vi "Shape Filter.vi"(11 "Image In":T1) -> (2 "Line Cam Obstacles":cluster{dbl[], dbl[], i32}, 3 "Image (out)":T1)   [LabVIEW 2011]
uses:
  <vilib>/vision/Pattern Matching.llb/IMAQ Curve Parameters.ctl
  <vilib>/vision/Analysis.llb/IMAQ ExtractCurvesCurve.ctl
  <vilib>/vision/Image Controls.llb/IMAQ Image.ctl
  <vilib>/vision/NI_Vision_Development_Module.lvlib
panel:
  out "Intensity Graph":dbl[][](graph)
  out "Curves":T2[](array[typedef]) {"Points"."Y" format="%.2f"; "Points"."X" format="%.2f"}
  out "Image out":T1(plugin-control)
  in  "Curve Parameters":T3={"Extraction Mode"=0, "Edge Threshold"=75, "Edge Filter Size"=1, "Min Length"=25, "Row Search Step Size"=15, "Col Search Step Size"=15, "Max Endpoint Gap"=10, "Closed"=FALSE, "Subpixel"=FALSE} {"Extraction Mode" items=["Normal", "Uniform Regions"]; "Edge Filter Size" items=["Fine", "Normal", "Contour Tracing"]; "Max Endpoint Gap" min=0; "Col Search Step Size" min=1 max=255 step=1; "Row Search Step Size" min=1 max=255 step=1; "Min Length" min=0; "Edge Threshold" min=1 max=350 step=1}
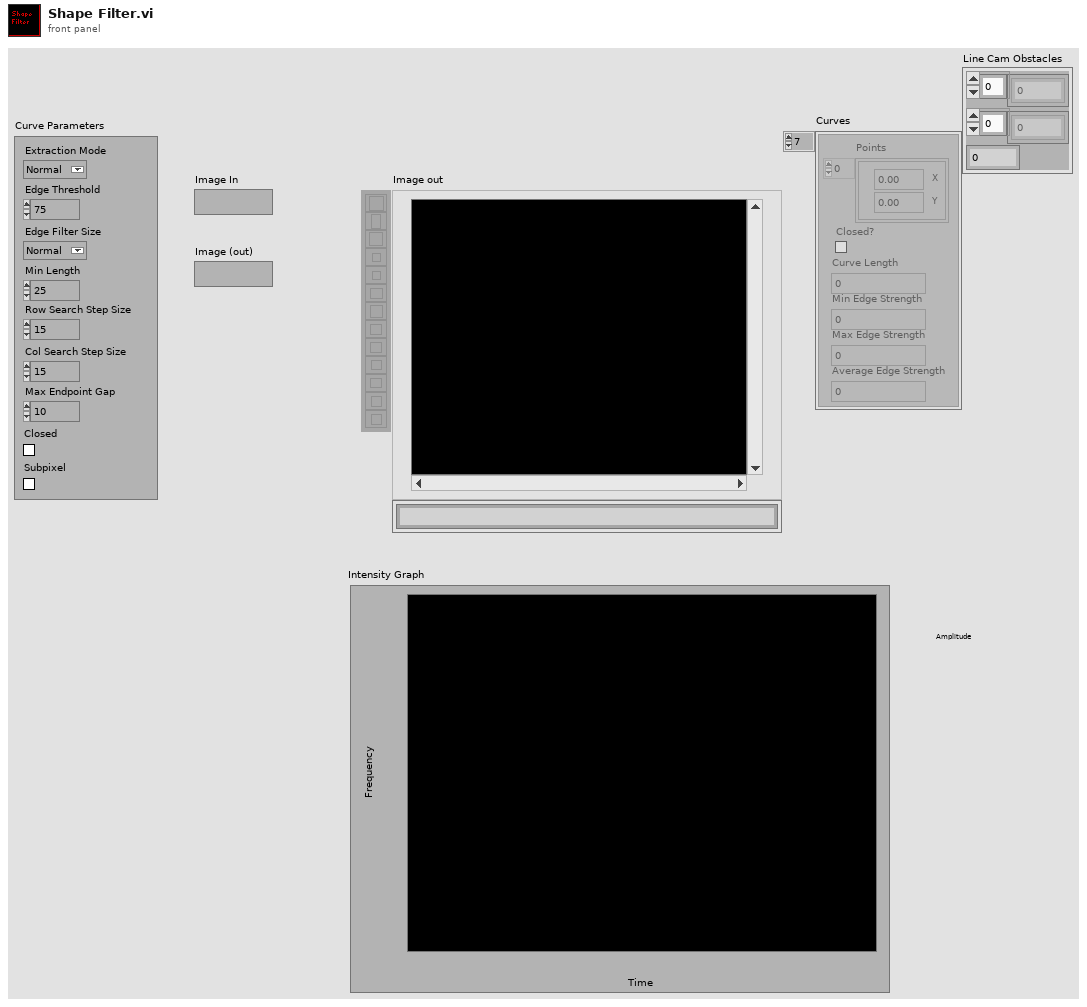
[diagram p1: front panel]
types:
  T1 = typedef "IMAQ Image.ctl" = refnum<image>
  T2 = typedef "IMAQ ExtractCurvesCurve.ctl" = cluster{"Points":cluster{"X":dbl, "Y":dbl}[], "Closed?":bool, "Curve Length":dbl, "Min Edge Strength":dbl, "Max Edge Strength":dbl, "Average Edge Strength":dbl}
  T3 = typedef "IMAQ Curve Parameters.ctl" = cluster{"Extraction Mode":u32, "Edge Threshold":i32, "Edge Filter Size":u32, "Min Length":i32, "Row Search Step Size":i32, "Col Search Step Size":i32, "Max Endpoint Gap":i32, "Closed":bool, "Subpixel":bool}
  T4 = typedef "Image Type" = u32
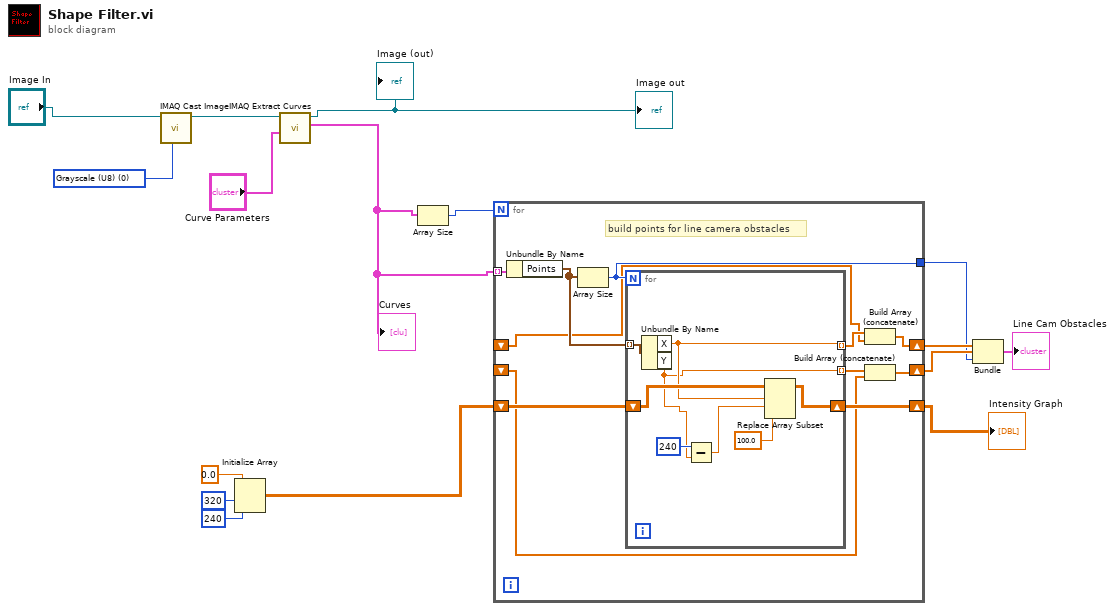
[diagram p0: block diagram]
diagram:
  w13 = T4 0 items=["Grayscale (U8)", "Grayscale (I16)", "Grayscale (SGL)", "Complex (CSG)", "RGB (U32)", "HSL (U32)", "RGB (U64)", "Grayscale (U16)"] ("Image Type")
  n1 = call "IMAQ Cast Image"("Image Type"=w13, "Image Src"="Image In") -> ("Image Dst Out"=w14:T1)  [unwired: 8 in, 1 out]
  n2 = Initialize Array(0.0 ("element"), 320 ("dimension size"), 240 ("dimension size")) -> (w8:dbl[][])
  n3 = call "IMAQ Extract Curves"("Curve Parameters"="Curve Parameters", "Image"=w14) -> ("Curves"=w7:T2[], "Image (dup)"=→"Image out" →"Image (out)":T1)  [unwired: 7 in, 1 out]
  "Curves" <- w7
  n4 = Array Size(array=w7) -> (size(s)=w12:i32)
  n5 = for {
    N: w12 -> [_]
    shift-right: [w25] -> w6
    shift-left: w8 -> [w26]
    tunnel: w7 -> [w27] mode=indexing
    tunnel: [w23] -> w2
    shift-right: [w21] -> w4
    shift-left: _ -> [w20]
    shift-right: [w18] -> w3
    shift-left: _ -> [w17]
    # "build points for line camera obstacles"
    n6 = Unbundle By Name(w27) -> ("Points"=w24:cluster{"X":dbl, "Y":dbl}[])
    n7 = Array Size(array=w24) -> (size(s)=w23:i32)
    n8 = for {
      N: w23 -> [_]
      shift-right: [w33] -> w25
      shift-left: w26 -> [w34]
      tunnel: w24 -> [w35] mode=indexing
      tunnel: [w29] -> w22 mode=indexing
      tunnel: [w28] -> w19 mode=indexing
      n9 = Unbundle By Name(w35) -> ("X"=w29:dbl, "Y"=w28:dbl)
      n10 = Subtract(x=240, y=w28) -> (x-y=w31:dbl)
      n11 = Replace Array Subset(array=w34, new element=100.0 ("element"), index (row)=w29, index (col)=w31) -> (w33:dbl[][])
    }
    n12 = Build Array (concatenate)(w22, w20) -> (w21:dbl[])
    n13 = Build Array (concatenate)(w19, w17) -> (w18:dbl[])
  }
  "Intensity Graph" <- w6
  n14 = Bundle(w4, w3, w2) -> (→"Line Cam Obstacles":cluster{dbl[], dbl[], i32})  [unwired: 1 in]
